vi "create dispatcher.vi"(8 "error in":errorcluster, 9 "default reporter":refnum<class "results reporter.lvclass">, 11 "initial pool sizes":T1) -> (0 "error out":errorcluster, 3 "dispatcher":refnum<data-value>)   [LabVIEW 2013, in "thread pool.lvclass"]
uses:
  thread pool.lvclass
  results reporter/results reporter.lvclass
  pool sizes.ctl
  thread pool.lvclass/thread pool.ctl
  task/task.lvclass
  standard reporters/event reporter/event reporter.lvclass
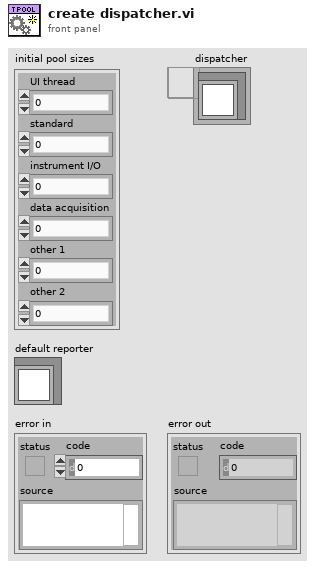
[diagram p1: front panel]
types:
  T1 = typedef "thread pool.lvclass/pool sizes.ctl" = cluster{"UI thread":u8, "standard":u8, "instrument I/O":u8, "data acquisition":u8, "other 1":u8, "other 2":u8}
  T2 = typedef "thread pool.lvclass/vi references.ctl" = cluster{"UI thread":T3, "standard":T3, "instrument I/O":T3, "data acquisition":T3, "other 1":T3, "other 2":T3}
  T3 = typedef "thread pool.lvclass/strict executor reference.ctl" = refnum<vi>
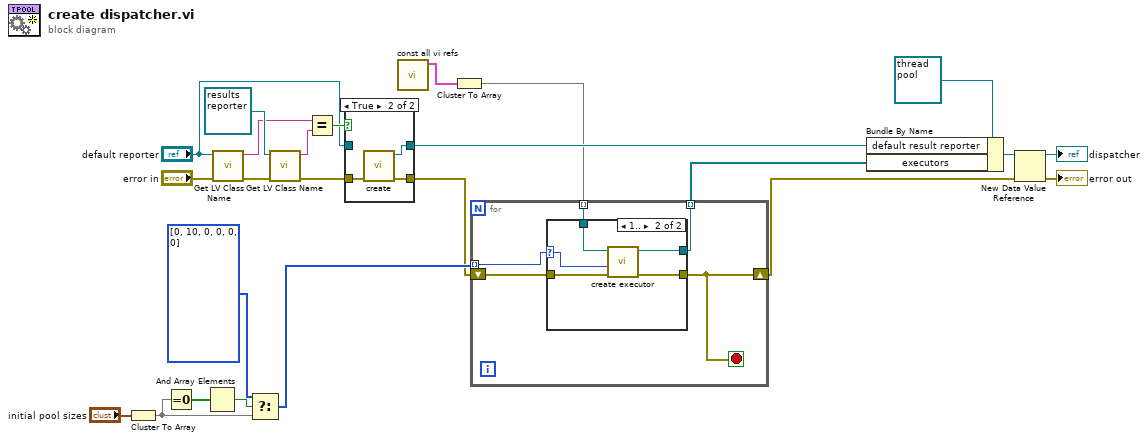
[diagram p0: block diagram]
diagram:
  n1 = Cluster To Array(cluster="initial pool sizes") -> (array=w8:u8[])
  n2 = Equal To 0?(x=w8) -> (x = 0?=w11:bool[])
  n3 = And Array Elements(Boolean array=w11) -> (logical AND=w10:bool)
  n4 = call <vilib>:"Get LV Class Name.vi"("error in (no error)"="error in", "object"="default reporter") -> ("error out"=w18:errorcluster, "class name"=w16:string)  [unwired: 8 in]
  n5 = Select(t=u8[] [0, 10, 0, 0, 0, 0] ("array"), s=w10, f=w8) -> (s? t:f=w6:u8[])
  n6 = call <vilib>:"Get LV Class Name.vi"("error in (no error)"=w18, "object"=refnum<class "results reporter.lvclass"> refnum ("results reporter")) -> ("error out"=w12:errorcluster, "class name"=w17:string)  [unwired: 8 in]
  n7 = Equal?(x=w16, y=w17) -> (x = y?=w15:bool)
  n8 = case shown="True" w15 {
    tunnel: "default reporter" -> [w26 _]
    tunnel: [w26 w27] -> w13
    tunnel: [w25 w28] -> w4
    tunnel: w12 -> [w25 w29]
    frame False {
    }
    frame True {
      n9 = call "create.vi"("error in"=w29) -> ("error out"=w28:errorcluster, "event reporter out"=w27:refnum<class "event reporter.lvclass">)  [unwired: 9 in]
    }
  }
  n10 = call "const all vi refs.vi"() -> ("initial pool sizes"=w2:T2)  [unwired: 11 in]
  n11 = Cluster To Array(cluster=w2) -> (array=w1:T3[])
  n12 = for {
    tunnel: w6 -> [w30] mode=indexing
    tunnel: [w34] -> w5 mode=indexing
    shift-right: [w32] -> w3
    shift-left: w4 -> [w33]
    tunnel: w1 -> [w31] mode=indexing
    stop <- w32 stop-if-true
    n13 = case shown="1.." w30 {
      selector: w30 -> [_ w36]
      tunnel: [_ w40] -> w34
      tunnel: w33 -> [w35 w39]
      tunnel: [w35 w38] -> w32
      tunnel: w31 -> [_ w37]
      frame ..0 {
      }
      frame 1.. {
        n14 = call "create executor.vi"("error in"=w39, "default pool size"=w36, "launcher ref"=w37) -> ("error out"=w38:errorcluster, "executor reference"=w40:T3)  [unwired: 7 in]
      }
    }
  }
  n15 = Bundle By Name(cluster=refnum<class "thread pool.lvclass"> refnum ("dispatcher.lvclass"), "default result reporter"=w13, "executors"=w5) -> (w22:refnum<class "thread pool.lvclass">)
  n16 = New Data Value Reference(data value=w22, error in=w3) -> (data value reference=→"dispatcher":refnum<data-value>, error out=→"error out":errorcluster)
